vi "Set Attributes.vi"(8 "error in (no error)":errorcluster, 11 "Test Step Dialog in":refnum<class "Test Step Dialog.lvclass">) -> (0 "error out":errorcluster, 3 "Test Step Dialog out":refnum<class "Test Step Dialog.lvclass">)   [LabVIEW 2017, in "Test Step Dialog.lvclass"]
uses:
  Test Step Dialog.lvclass
  ITest Executive Builder Dialog/ITest Executive Builder Dialog.lvclass
  <vilib>/gpm_packages/@cs/test-executive/Source/Test Executive/TestExecutive Ref/TestExecutive Ref.lvclass
  fc07f503-8f6a-4dc4-9222-dc8448c3f596.vi
  4943faeb-c81e-4e0c-b9cd-ea5a5410b3bf.vi
  40a32776-d461-4076-ab80-029c81831e6c.vi
  C:/Users/jonmc/Documents/Git/Test Executive Builder/Source/Test Executive Builder Dialogs/ITest Executive Builder Dialog/ITest Executive Builder Dialog.lvclass
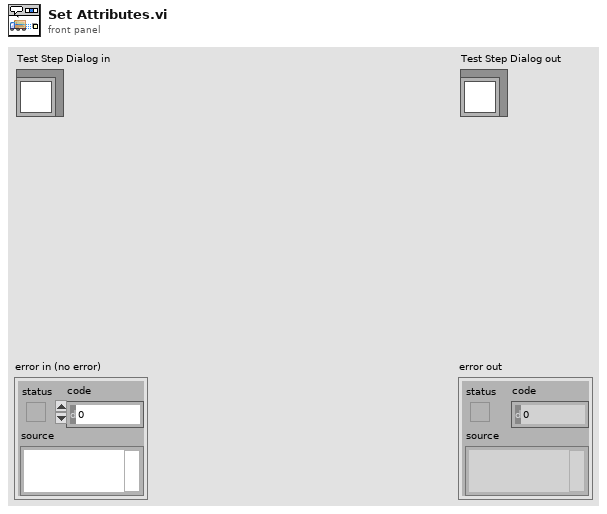
[diagram p1: front panel]
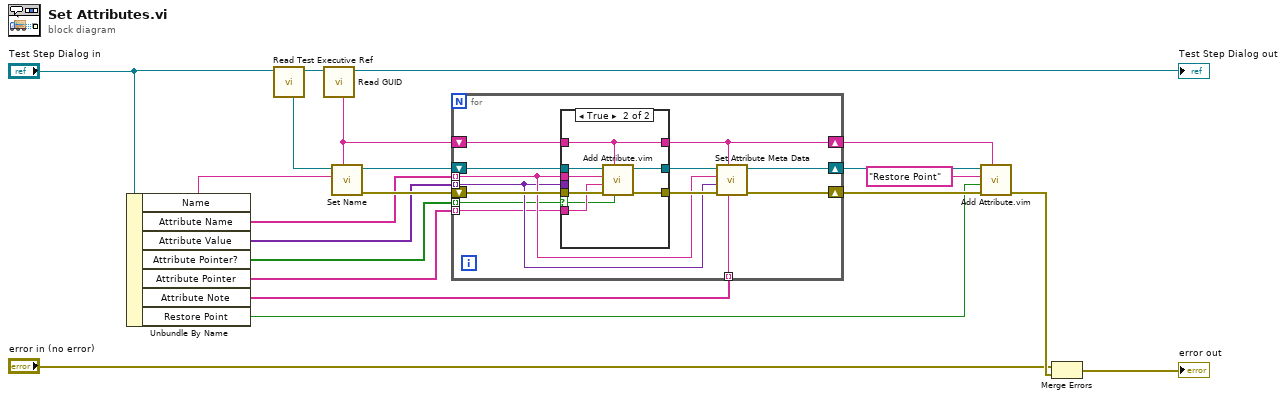
[diagram p0: block diagram]
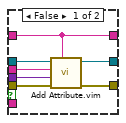
[diagram p2: hidden frame]
diagram:
  n1 = Unbundle By Name("Test Step Dialog in") -> ("Name"=w19:string, "Attribute Name"=w6:string[], "Attribute Value"=w7:variant[], "Attribute Pointer?"=w8:bool[], "Attribute Pointer"=w9:string[], "Attribute Note"=w10:string[], "Restore Point"=w11:bool)
  n2 = call "Read Test Executive Ref.vi"("ITest Executive Builder Dialog in"="Test Step Dialog in") -> ("ITest Executive Builder Dialog out"=w21:refnum<class "Test Step Dialog.lvclass">, "Test Executive Ref"=w20:refnum<data-value>)  [unwired: 9 in]
  n3 = call "Read GUID.vi"("ITest Executive Builder Dialog in"=w21) -> ("ITest Executive Builder Dialog out"=→"Test Step Dialog out":refnum<class "Test Step Dialog.lvclass">, "GUID"=w12:string)  [unwired: 9 in]
  n4 = call <vilib>:"Set Name.vi"("Unique ID"=w12, "Name"=w19, "Test Executive Ref"=w20) -> ("error out"=w13:errorcluster, "Test Executive Ref out"=w14:refnum<data-value>)  [unwired: 7 in]
  n5 = for {
    shift-right: [w31] -> w16
    shift-left: w14 -> [w34]
    shift-right: [w29] -> w15
    shift-left: w13 -> [w33]
    tunnel: w6 -> [w27] mode=indexing
    tunnel: w7 -> [w26] mode=indexing
    shift-right: [w22] -> w17
    shift-left: w12 -> [w25]
    tunnel: w10 -> [w28] mode=indexing
    tunnel: w8 -> [w24] mode=indexing
    tunnel: w9 -> [w23] mode=indexing
    n6 = case shown="True" w24 {
      selector: w24 -> [_ w42]
      tunnel: w34 -> [w41 w49]
      tunnel: w33 -> [w40 w48]
      tunnel: [w39 w47] -> w32
      tunnel: [w38 w46] -> w30
      tunnel: w27 -> [w37 w45]
      tunnel: w26 -> [w36 _]
      tunnel: w25 -> [w35 w44]
      tunnel: w23 -> [_ w43]
      tunnel: [w35 w44] -> w22
      frame False {
        n7 = call "Add Attribute.vim"("ID"=w35, "error in (no error)"=w40, "Attribute"=w36, "Attribute Name"=w37, "Test Executive Ref"=w41) -> ("error out"=w38:errorcluster, "Test Executive Ref out"=w39:refnum<data-value>)  [unwired: 3 in, 2 out]
      }
      frame True {
        n8 = call "Add Attribute.vim"("Pointer?"=w42, "ID"=w44, "error in (no error)"=w48, "Attribute"=w43, "Attribute Name"=w45, "Test Executive Ref"=w49) -> ("error out"=w46:errorcluster, "Test Executive Ref out"=w47:refnum<data-value>)  [unwired: 2 in, 2 out]
      }
    }
    n9 = call <vilib>:"Set Attribute Meta Data.vi"("Meta Data"=w28, "Unique ID"=w22, "error in (no error)"=w30, "Attribute Type"=w26, "Attribute Name"=w27, "Test Executive Ref"=w32) -> ("error out"=w29:errorcluster, "Test Executive Ref out"=w31:refnum<data-value>)  [unwired: 3 in, 1 out]
  }
  n10 = call "Add Attribute.vim"("ID"=w17, "error in (no error)"=w15, "Attribute"=w11, "Attribute Name"="Restore Point", "Test Executive Ref"=w16) -> ("error out"=w5:errorcluster)  [unwired: 3 in, 3 out]
  n11 = Merge Errors("error in (no error)", w5) -> (→"error out":errorcluster)
